vi "InitSerialPort.vi"(1 "default resource name":refnum<visa-resource-name>) -> (0 "VISA resource name out":refnum<visa-resource-name>)   [LabVIEW 2010]
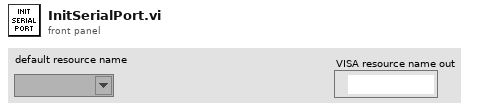
[diagram p1: front panel]
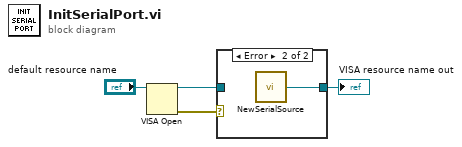
[diagram p0: block diagram]
diagram:
  n1 = VISA Open(VISA resource name="default resource name") -> (VISA resource name=w2:refnum<visa-resource-name>, error out=w1:errorcluster)  [unwired: 4 in]
  n2 = case shown="Error" w1 {
    tunnel: [w5 w6] -> w3
    tunnel: w2 -> [w5 _]
    frame No Error {
    }
    frame Error {
      n3 = call "NewSerialSource.vi"() -> ("Select Source 2"=w6:refnum<visa-resource-name>)  [unwired: 1 in]
    }
  }
  "VISA resource name out" <- w3
